vi "Set Report Font.vi"(0 "report in":refnum<class "NI_Standard Report.lvclass">, 1 "text color (unchanged)":u32(colorbox)=16777216, 2 "font settings source":u16(ring) items=["VI Inputs", "Font Dialog Box"], 5 "text options":T2, 9 "font settings":T3={"Charset (-1)"=-1, "Weight (-1)"=-1, "Name"="", "Size"=" "}, 11 "error in (no error)":errorcluster) -> (4 "report out":refnum<class "NI_Standard Report.lvclass">, 6 "font out":T1={"font name"="", "font size"=0.0, "bold"=0, "italic"=0, "underline"=0, "strike through"=0, "font color"=16777216} {"font size" format="%0.2f"; "strike through" items=["Unchanged", "Yes", "No"]; "underline" items=["Unchanged", "Yes", "No"]; "italic" items=["Unchanged", "Yes", "No"]; "bold" items=["Unchanged", "Yes", "No"]}, 15 "error out":errorcluster)   [LabVIEW 2017, in "NI_Standard Report.lvclass"]
doc: "Sets the font properties of the report, including those in the headers and footers."
uses:
  <vilib>/Utility/NIReport.llb/Standard Report/NI_Standard Report.lvclass
  <vilib>/Utility/NIReport.llb/font.ctl
  <vilib>/Utility/NIReport.llb/Standard Report/NI_Standard Report.lvclass/NI_Standard Report.ctl
  <vilib>/Utility/NIReport.llb/NI_ReportGenerationCore.lvlib
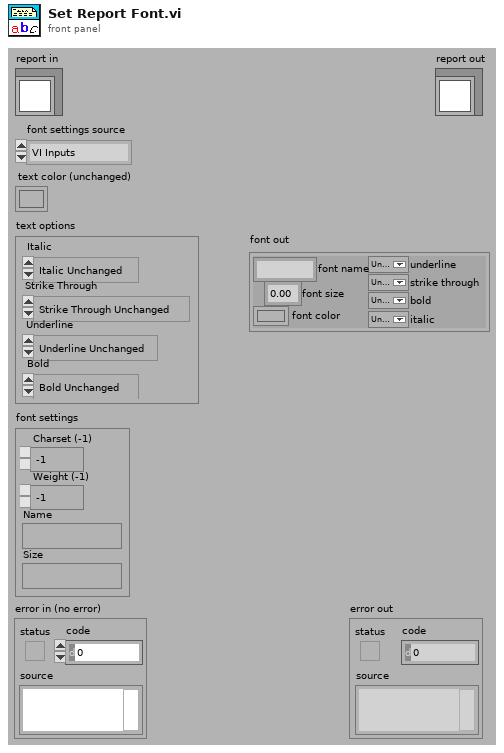
[diagram p1: front panel]
types:
  T1 = typedef "NI_ReportGenerationCore.lvlib/font.ctl" = cluster{"font name":string, "font size":dbl, "bold":u16, "italic":u16, "underline":u16, "strike through":u16, "font color":u32}
  T2 = cluster{"Italic":enum16{"Italic Unchanged", "Italic On", "Italic Off"}, "Strike Through":enum16{"Strike Through Unchanged", "Strike Through On", "Strike Through Off"}, "Underline":enum16{"Underline Unchanged", "Underline On", "Underline Off"}, "Bold":enum16{"Bold Unchanged", "Bold On", "Bold Off"}}
  T3 = cluster{"Charset (-1)":i16, "Weight (-1)":i16, "Name":string, "Size":string}
  T4 = typedef "NI_ReportGenerationCore.lvlib/Report Data Members.ctl" = cluster{"font":T1, "from template?":bool}
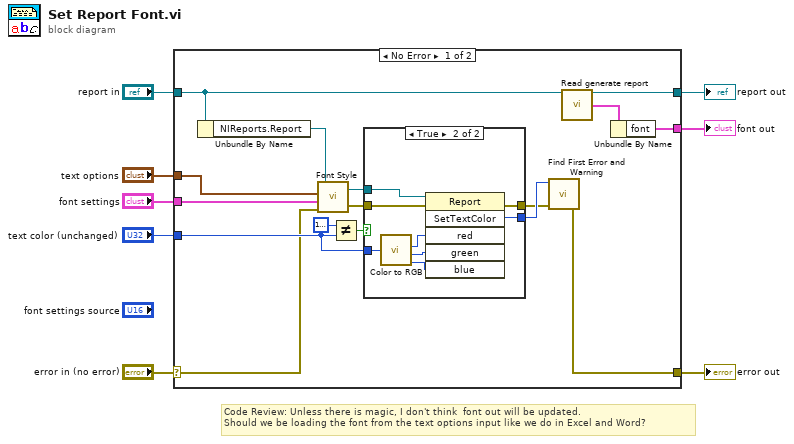
[diagram p0: block diagram]
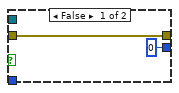
[diagram p2: hidden frame]
diagram:
  # "Code Review: Unless there is magic, I don't think  font out will be updated.  \nShould we be loading the font from the text options input like we do in Excel and Word?"
  n1 = case shown="No Error" "error in (no error)" {
    selector: "error in (no error)" -> [w14 w36]
    tunnel: [w13 w36] -> w7
    tunnel: [w9 w35] -> w5
    tunnel: "report in" -> [w10 w35]
    tunnel: "text options" -> [w17 _]
    tunnel: "font settings" -> [w16 _]
    tunnel: "text color (unchanged)" -> [w15 _]
    tunnel: [w12 _] -> w1
    frame No Error {
      n2 = Unbundle By Name(w10) -> ("NIReports.Report"=w24:refnum<k7>)
      n3 = call <vilib>:"Font Style.vi"("error in (no error)"=w14, "Font Settings"=w16, "Text Options"=w17, "NIReports.Report"=w24) -> ("error out"=w20:errorcluster, "NIReports.Report out"=w21:refnum<k7>)
      n4 = Not Equal?(x=u32 16777216, y=w15) -> (x != y?=w19:bool)
      n5 = case shown="True" w19 {
        tunnel: [0 ("SetTextColor") w33] -> w23
        tunnel: w20 -> [w25 w32]
        tunnel: w21 -> [_ w31]
        tunnel: [w25 w34] -> w22
        tunnel: w15 -> [_ w27]
        frame False {
        }
        frame True {
          n6 = call <vilib>:"Color to RGB.vi"("Color"=w27) -> ("R"=w29:u8, "G"=w30:u8, "B"=w28:u8)  [unwired: 1 out]
          n7 = invoke class="Report" method="SetTextColor"(reference=w31, error in=w32, "red"=w29, "green"=w30, "blue"=w28) -> (error out=w34:errorcluster, "SetTextColor"=w33:i32)  [unwired: 1 in, 4 out]
        }
      }
      n8 = call <vilib>:"Find First Error and Warning.vi"("error in (no error)"=w22, "error code"=w23) -> ("error out"=w13:errorcluster)  [unwired: 1 in, 4 out]
      n9 = call-dynamic "Read generate report.vi"("report in"=w10) -> ("report out"=w9:refnum<class "NI_Standard Report.lvclass">, "generate report"=w11:T4)  [unwired: 1 in, 12 out]
      n10 = Unbundle By Name(w11) -> ("font"=w12:T1)
    }
    frame Error {
    }
  }
  "error out" <- w7
  "report out" <- w5
  "font out" <- w1
